vi "Documentation Page.vi"() -> ()   [LabVIEW 2020, in "2D Plot.lvclass"]
uses:
  <vilib>/Math Plots/2D Math Plots/2D Plot/2D Plot/2D Plot.lvclass
  <vilib>/Math Plots/2D Math Plots/2D Plot/Action String/2DMathPlot Ctrl Act Queue.ctl
  <vilib>/Math Plots/2D Math Plots/2D Plot/Action String/2DMathPlot Ctrl Act Cluster.ctl
  <vilib>/Math Plots/2D Math Plots/2D Plot/Action String/2DMathPlot State Class.ctl
  <vilib>/Math Plots/2D Math Plots/2D Plot/2D Plot/Typedef/Dialog State.ctl
panel:
  in  "Event Registration":refnum<event-registration>
  in  "Control Ref Queue":T1
  in  "Tip strip":string
  in  "Description":string
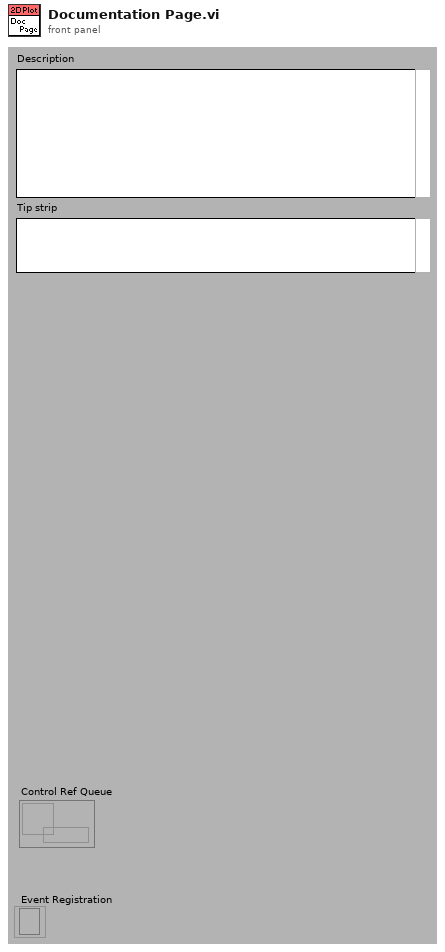
[diagram p1: front panel]
types:
  T1 = typedef "2DMathPlot Ctrl Act Queue.ctl" = refnum<queue>
  T2 = typedef "2D Plot.lvclass/Dialog State.ctl" = enum16{"Initialize", "Read Property", "Write Property", "Idle", "Exit"}
  T3 = typedef "2DMathPlot Ctrl Act Cluster.ctl" = cluster{"Plot Area Ref":refnum<vi>, "Z Axis Ref":refnum<vi>, "Legend Ref":refnum<vi>, "XControl Ref":refnum<vi>, "Facade Ref":refnum<vi>, "Display State Change Class":T4}
  T4 = typedef "2DMathPlot State Class.ctl" = enum16{"Update All (Undo)", "Update General", "Update Appearance", "Update Format", "Update Scale", "Update Marker", "Update Cursor", "None"}
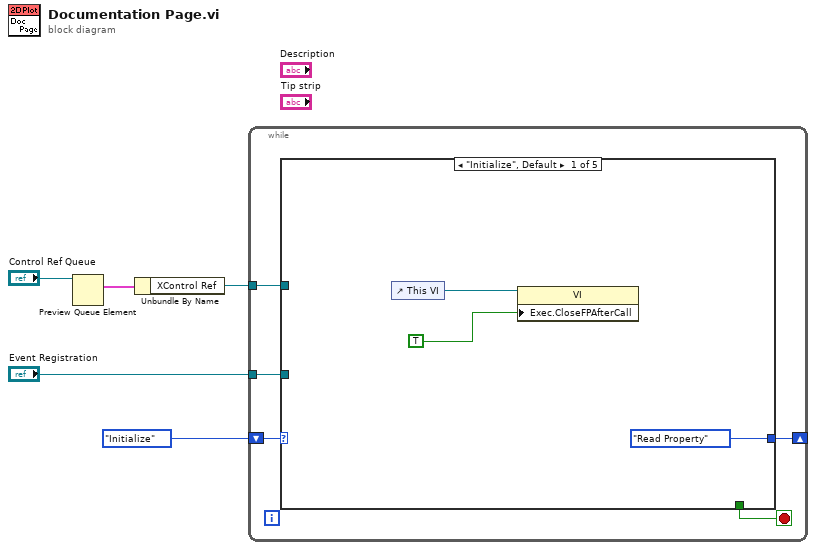
[diagram p0: block diagram]
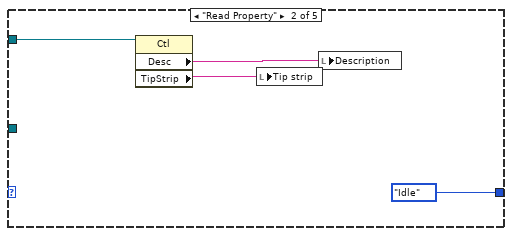
[diagram p2: hidden frame]
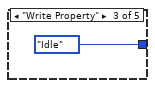
[diagram p3: hidden frame]
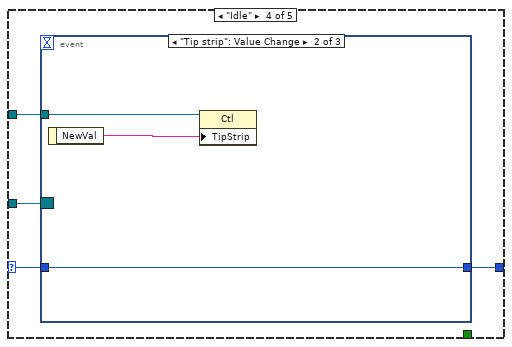
[diagram p4: hidden frame]
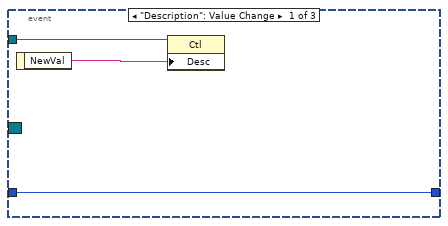
[diagram p5: hidden frame]
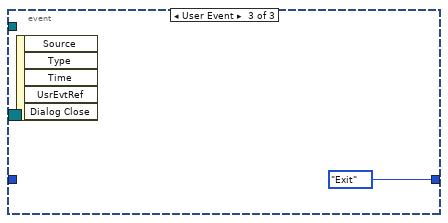
[diagram p6: hidden frame]
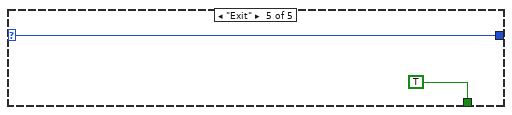
[diagram p7: hidden frame]
diagram:
  n1 = Preview Queue Element(queue="Control Ref Queue") -> (element=w4:T3)  [unwired: 1 in, 4 out]
  n2 = Unbundle By Name(w4) -> ("XControl Ref"=w2:refnum<vi>)
  n3 = while {
    shift-right: [w9] -> _
    shift-left: Dialog_State."Initialize" ("Enum") -> [w10]
    tunnel: w2 -> [w8]
    tunnel: "Event Registration" -> [w7]
    stop <- w6 stop-if-true
    n4 = case shown="\"Initialize\", Default" w10 {
      selector: w10 -> [_ _ _ w19 w31]
      tunnel: [Dialog_State."Read Property" ("Enum") Dialog_State."Idle" ("Enum") Dialog_State."Idle" ("Enum") w20 w31] -> w9
      tunnel: w8 -> [_ w17 _ w22 _]
      tunnel: w7 -> [_ _ _ w21 _]
      tunnel: [_ _ _ _ TRUE] -> w6
      frame "Initialize", Default {
        n5 = control-ref of="This VI"() -> (w11:refnum<vi>)
        n6 = property class="VI"(reference=w11, "Exec.CloseFPAfterCall"=TRUE ("Execution:Close After Call")) -> ()  [unwired: 1 in, 2 out]
      }
      frame "Read Property" {
        n7 = property class="Ctl"(reference=w17) -> ("Desc"=w15:string, "TipStrip"=w16:string)  [unwired: 1 in, 2 out]
        n8 = local write "Tip strip"(w16) -> ()
        n9 = local write "Description"(w15) -> ()
      }
      frame "Write Property" {
      }
      frame "Idle" {
        n10 = event shown="[1] \"Tip strip\": Value Change" {
          selector: w21 -> [_ _ _]
          dyn-events: _ -> [_ _ _]
          timeout: _ -> [_ _ _]
          tunnel: w22 -> [w25 w28 _]
          tunnel: [w23 w26 Dialog_State."Exit" ("Enum")] -> w20
          tunnel: w19 -> [w23 w26 _]
          event "Description": Value Change {
            n11 = event-data() -> ("NewVal"=w24:string)  [unwired: 1 out]
            n12 = property class="Ctl"(reference=w25, "Desc"=w24) -> ()  [unwired: 1 in, 2 out]
          }
          event "Tip strip": Value Change {
            n13 = event-data() -> ("NewVal"=w27:string)  [unwired: 1 out]
            n14 = property class="Ctl"(reference=w28, "TipStrip"=w27) -> ()  [unwired: 1 in, 2 out]
          }
          event User Event {
            n15 = event-data() -> ()  [unwired: 6 out]
          }
        }
      }
      frame "Exit" {
      }
    }
  }
